vi "_ValidateDeviceProfiles.vi"(8 "error in (no error)":errorcluster, 9 "ddSrcPath":string[](array[string]), 10 "reference in":refnum<vi>) -> (0 "error out":errorcluster, 1 "profileImport":T1[](array[typedef]), 2 "reference out":refnum<vi>)   [LabVIEW 2019, in "SEECD System Explorer.lvlib"]
uses:
  SEECD System Explorer.lvlib
  <resource>/Framework/Providers/indcomecat/_InternalSubVIs/_profileImport.ctl
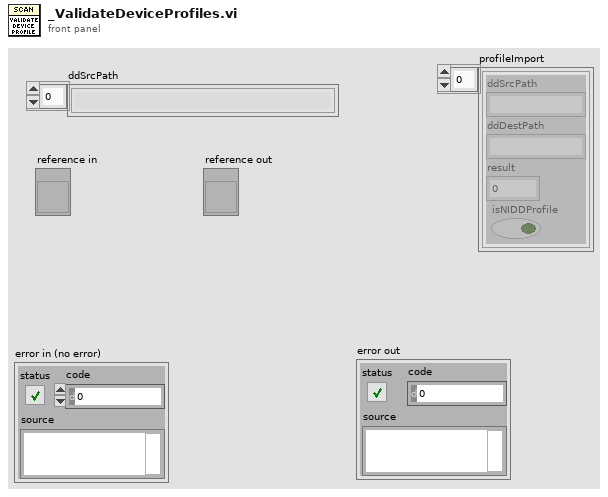
[diagram p1: front panel]
types:
  T1 = typedef "_profileImport.ctl" = cluster{"ddSrcPath":string, "ddDestPath":string, "result":i32, "isNIDDProfile":bool}
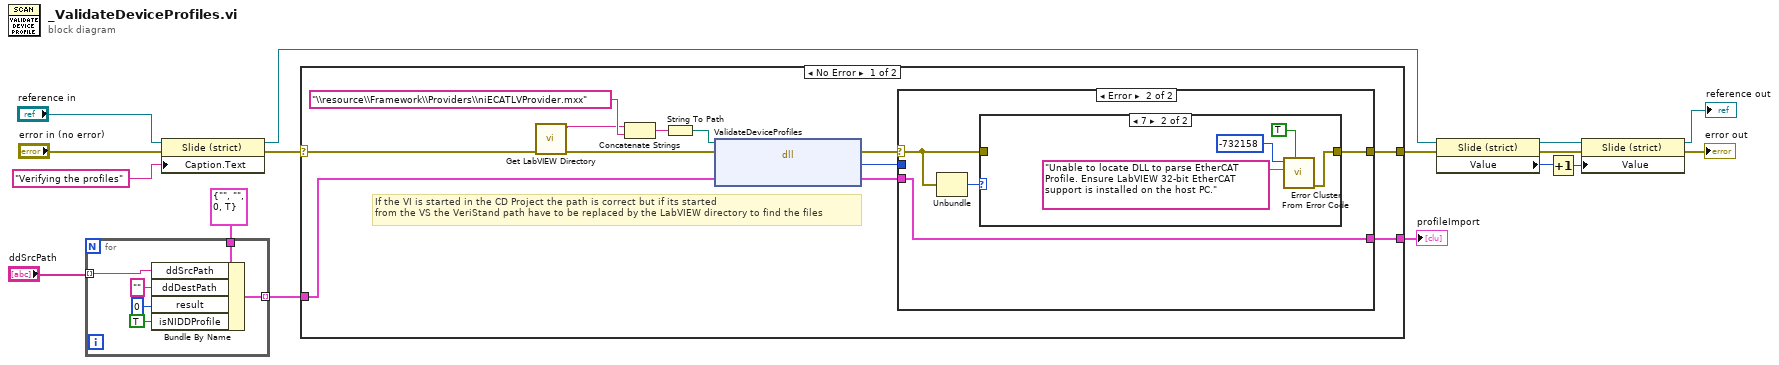
[diagram p0: block diagram]
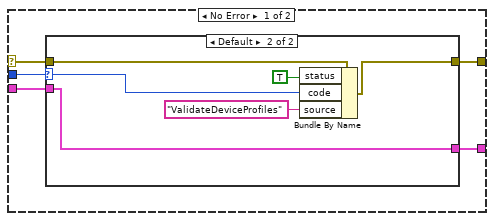
[diagram p2: hidden frame]
diagram:
  n1 = for {
    tunnel: "ddSrcPath" -> [w21] mode=indexing
    tunnel: [w22] -> w14 mode=indexing
    tunnel: T1 {"ddSrcPath"="", "ddDestPath"="", "result"=0, "isNIDDProfile"=TRUE} ("input cluster") -> [w20]
    n2 = Bundle By Name(cluster=w20, "ddSrcPath"=w21, "ddDestPath"="" ("ddRootPath"), "result"=0, "isNIDDProfile"=TRUE) -> (w22:T1)
  }
  n3 = property class="Slide (strict)"(reference="reference in", error in="error in (no error)", "Caption.Text"="Verifying the profiles") -> (reference out=w1:refnum<vi>, error out=w11:errorcluster)
  n4 = case shown="No Error" w11 {
    selector: w11 -> [w25 w58]
    tunnel: [w32 w58] -> w8
    tunnel: w14 -> [w29 w57]
    tunnel: [w30 w57] -> w13
    frame No Error {
      # "If the VI is started in the CD Project the path is correct but if its started \nfrom the VS the VeriStand path have to be replaced by the LabVIEW directory to find the files"
      n5 = call "Get LabVIEW Directory.vi"("error in"=w25) -> ("error out"=w24:errorcluster, "LabVIEW Directory"=w23:string)  [unwired: 9 in]
      n6 = Concatenate Strings(w23, "\\resource\\Framework\\Providers\\niECATLVProvider.mxx") -> (w27:string)
      n7 = String To Path(string=w27) -> (path=w26:path)
      n8 = dll-call lib="C:/Users/grschero/Desktop/CD-Project Folder/CD_Project/Scan-Engine-Custom-Device_EtherCAT_AKD_Extension/Scan-Engine-Custom-Device/Custom Device Source/niECATLVProvider.mxx" fn="ValidateDeviceProfiles"(path in=w26, error in=w24, "profileImport"=w29) -> (error out=w31:errorcluster, "return type"=w33:i32, "profileImport"=w34:T1[])  [unwired: 1 in, 1 out]
      n9 = case shown="Error" w31 {
        selector: w31 -> [w36 w49]
        tunnel: w34 -> [w39 w51]
        tunnel: w33 -> [w38 _]
        tunnel: [w37 w48] -> w32
        tunnel: [w35 w51] -> w30
        frame No Error {
          n10 = case shown="Default" w38 {
            selector: w38 -> [_ w47]
            tunnel: [w41 w44] -> w37
            tunnel: w36 -> [w41 w43]
            tunnel: w39 -> [w40 w42]
            tunnel: [w40 w42] -> w35
            frame 0 {
            }
            frame Default {
              n11 = Bundle By Name(cluster=w43, "status"=TRUE, "code"=w47, "source"="ValidateDeviceProfiles") -> (w44:errorcluster)
            }
          }
        }
        frame Error {
          n12 = Unbundle(w49) -> ("code"=w50:i32)  [unwired: 2 out]
          n13 = case shown="7" w50 {
            tunnel: w49 -> [w52 _]
            tunnel: [w52 w56] -> w48
            frame Default {
            }
            frame 7 {
              n14 = call <vilib>:"Error Cluster From Error Code.vi"("show call chain? (False)"=TRUE, "error message (\"\")"="Unable to locate DLL to parse EtherCAT Profile. Ensure LabVIEW 32-bit EtherCAT support is installed on the host PC." ("error message (\"\")"), "error code (0)"=-732158) -> ("error out"=w56:errorcluster)  [unwired: 6 in]
            }
          }
        }
      }
    }
    frame Error {
    }
  }
  "profileImport" <- w13
  n15 = property class="Slide (strict)"(reference=w1, error in=w8) -> (reference out=w4:refnum<vi>, error out=w5:errorcluster, "Value"=w7:u8)
  n16 = Increment(x=w7) -> (x+1=w6:u8)
  n17 = property class="Slide (strict)"(reference=w4, error in=w5, "Value"=w6) -> (reference out=→"reference out":refnum<vi>, error out=→"error out":errorcluster)
